vi "build-filepath.vi"(8 "Include Seconds in Filename":bool, 11 "Log Filepath Selection":T1={"Log Filepath Source"=enum."Application Relative (Auto)", "Log File Path (Manual)"=path "C:/Users/dheard/Documents/0002-labview-projects/ammonia-absorbsion-rig/data", "Log File Folder Name"="data", "log file name"="log", "Include Date in Filename"=TRUE, "Include Time in Filename"=TRUE}) -> (3 "appended path for log file":path, 5 "date string":string)   [LabVIEW 2024]
uses:
  filepath-selection.ctl
panel:
  out "Application Directory":path
  out "datetime-mode":u32
  out "log folder path":path
  out "stripped path":path
  out "vi path":path
  # "Filepath"
  # "File Name"
  # "Auto Generation"
  # "Path is relative to application or VI"
  # "Path Stripped to Local Directory"
  # "This will be the path log files are saved to"
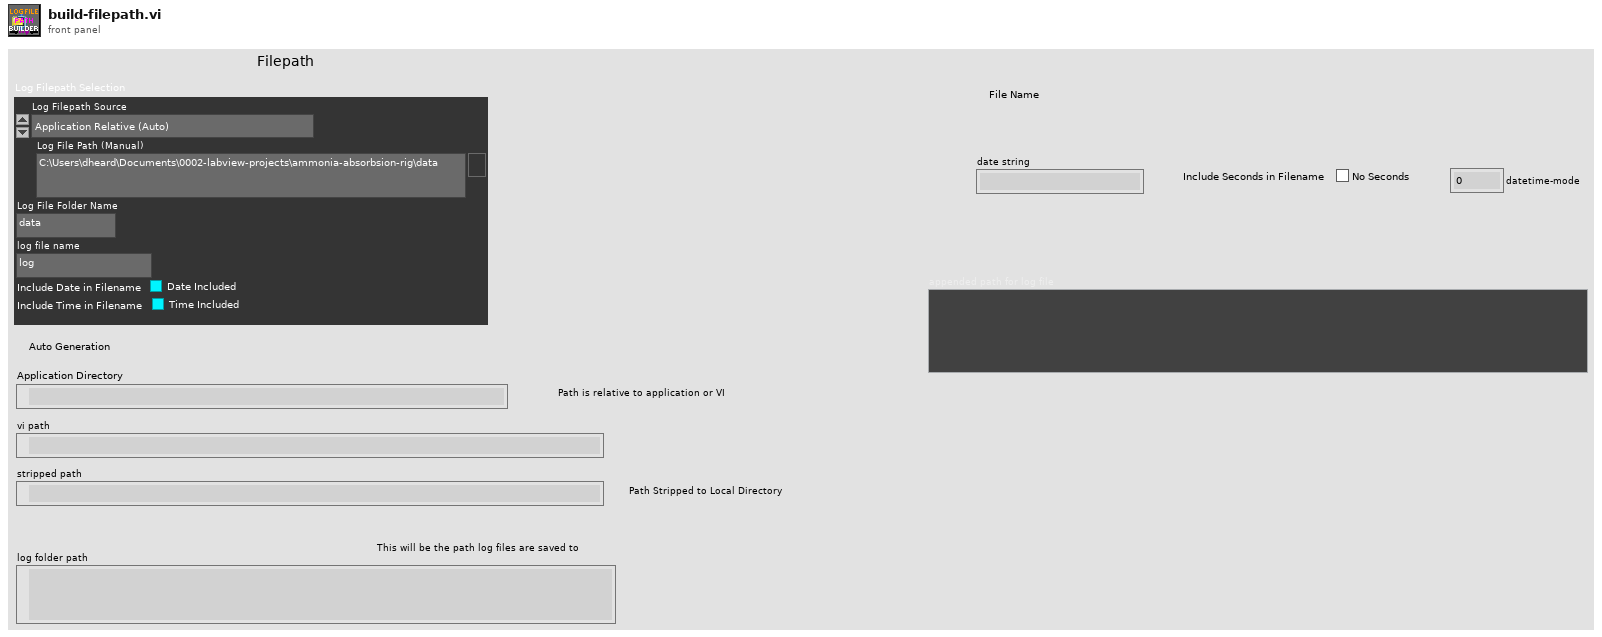
[diagram p1: front panel]
types:
  T1 = typedef "filepath-selection.ctl" = cluster{"Log Filepath Source":enum16{"Application Relative (Auto)", "VI Relative (Auto)", "Complete Path (Manual)"}, "Log File Path (Manual)":path, "Log File Folder Name":string, "log file name":string, "Include Date in Filename":bool, "Include Time in Filename":bool}
  T2 = enum16{"Application Relative (Auto)", "VI Relative (Auto)", "Complete Path (Manual)"}
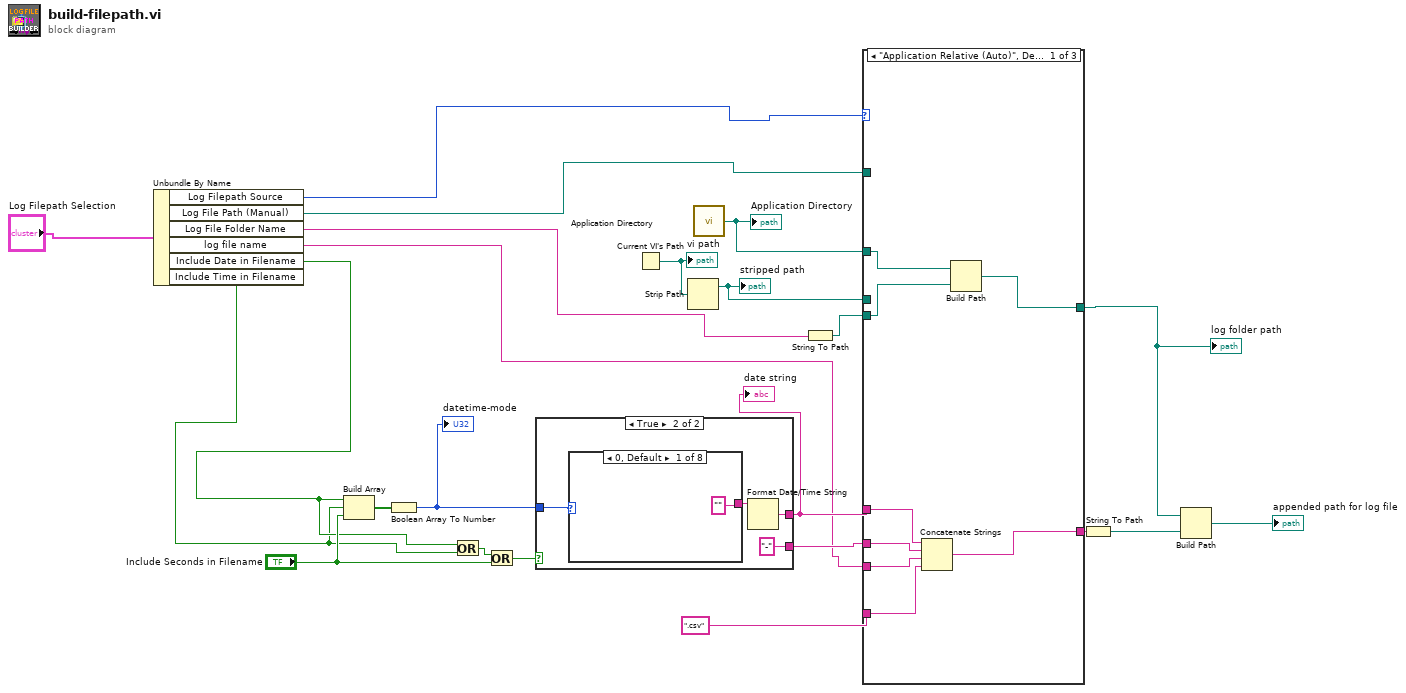
[diagram p0: block diagram]
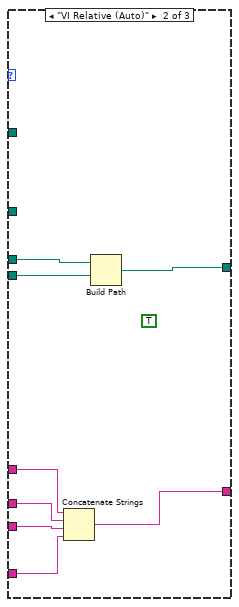
[diagram p2: hidden frame]
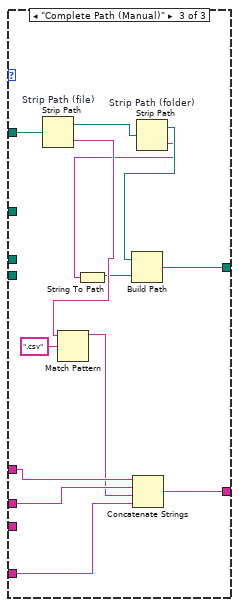
[diagram p3: hidden frame]
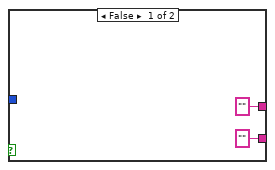
[diagram p4: hidden frame]
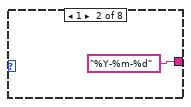
[diagram p5: hidden frame]
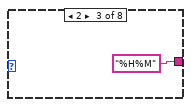
[diagram p6: hidden frame]
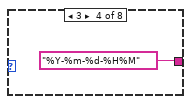
[diagram p7: hidden frame]
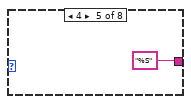
[diagram p8: hidden frame]
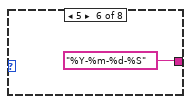
[diagram p9: hidden frame]
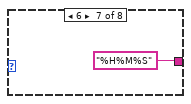
[diagram p10: hidden frame]
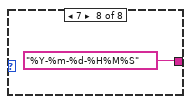
[diagram p11: hidden frame]
diagram:
  n1 = Unbundle By Name("Log Filepath Selection") -> ("Log Filepath Source"=w7:T2, "Log File Path (Manual)"=w6:path, "Log File Folder Name"=w5:string, "log file name"=w2:string, "Include Date in Filename"=w4:bool, "Include Time in Filename"=w3:bool)
  n2 = Build Array(w4, w3, "Include Seconds in Filename") -> (w19:bool[])
  n3 = Boolean Array To Number(Boolean array=w19) -> (number=w23:u32)
  "datetime-mode" <- w23
  n4 = Or(x=w4, y=w3) -> (x .or. y?=w20:bool)
  n5 = Or(x=w20, y="Include Seconds in Filename") -> (x .or. y?=w21:bool)
  n6 = case shown="True" w21 {
    tunnel: ["" ("date/time string") w29] -> w13
    tunnel: w23 -> [_ w27]
    tunnel: ["" ("string") "-" ("string")] -> w12
    frame False {
    }
    frame True {
      n7 = case shown="0, Default" w27 {
        tunnel: ["" ("time format string (%c)") "%Y-%m-%d" ("time format string (%c)") "%H%M" ("time format string (%c)") "%Y-%m-%d-%H%M" ("time format string (%c)") "%S" ("time format string (%c)") "%Y-%m-%d-%S" ("time format string (%c)") "%H%M%S" ("time format string (%c)") "%Y-%m-%d-%H%M%S" ("time format string (%c)")] -> w28
        frame 0, Default {
        }
        frame 1 {
        }
        frame 2 {
        }
        frame 3 {
        }
        frame 4 {
        }
        frame 5 {
        }
        frame 6 {
        }
        frame 7 {
        }
      }
      n8 = Format Date/Time String(time format string (%c)=w28) -> (date/time string=w29:string)  [unwired: 2 in]
    }
  }
  "date string" <- w13
  n9 = Current VI's Path() -> (path=w16:path)
  "vi path" <- w16
  n10 = Strip Path(path=w16) -> (stripped path=w15:path)  [unwired: 1 out]
  "stripped path" <- w15
  n11 = call <vilib>:"Application Directory.vi"() -> ("Application Directory"=w14:path)
  "Application Directory" <- w14
  n12 = String To Path(string=w5) -> (path=w8:path)
  n13 = case shown="\"Application Relative (Auto)\", Default" w7 {
    tunnel: w15 -> [_ w48 _]
    tunnel: w14 -> [w40 _ _]
    tunnel: w6 -> [_ _ w62]
    tunnel: w13 -> [w42 w52 w64]
    tunnel: w12 -> [w43 w51 w66]
    tunnel: w2 -> [w45 w50 _]
    tunnel: ".csv" ("string") -> [w44 w49 w63]
    tunnel: [w41 w53 w65] -> w10
    tunnel: [w39 w47 w61] -> w9
    tunnel: w8 -> [w38 w46 _]
    frame "Application Relative (Auto)", Default {
      n14 = Concatenate Strings(w42, w43, w45, w44) -> (w41:string)
      n15 = Build Path(base path=w40, name or relative path=w38) -> (appended path=w39:path)
    }
    frame "VI Relative (Auto)" {
      (unwired) TRUE
      n16 = Concatenate Strings(w52, w51, w50, w49) -> (w53:string)
      n17 = Build Path(base path=w48, name or relative path=w46) -> (appended path=w47:path)
    }
    frame "Complete Path (Manual)" {
      n18 = Strip Path "Strip Path (file)"(path=w62) -> (stripped path=w57:path, name=w60:string)
      n19 = Match Pattern(string=w60, regular expression=".csv") -> (before substring=w58:string)  [unwired: 1 in, 3 out]
      n20 = Concatenate Strings(w64, w66, w58, w63) -> (w65:string)
      n21 = Strip Path "Strip Path (folder)"(path=w57) -> (stripped path=w56:path, name=w54:string)
      n22 = String To Path(string=w54) -> (path=w55:path)
      n23 = Build Path(base path=w56, name or relative path=w55) -> (appended path=w61:path)
    }
  }
  "log folder path" <- w9
  n24 = String To Path(string=w10) -> (path=w18:path)
  n25 = Build Path(base path=w9, name or relative path=w18) -> (appended path=→"appended path for log file":path)
